vi "Open Channel.vi"(6 "Open All (False)":bool, 7 "Channel List":string, 8 "error in (no error)":errorcluster, 11 "VISA resource name":refnum<visa-resource-name>) -> (0 "error out":errorcluster, 3 "VISA resource name out":refnum<visa-resource-name>)   [LabVIEW 2018, in "Keithley 3706.lvlib"]
uses:
  <instrlib>/Keithley 3706/Keithley 3706.lvlib
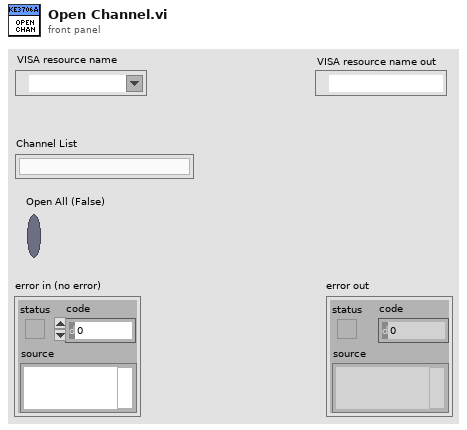
[diagram p1: front panel]
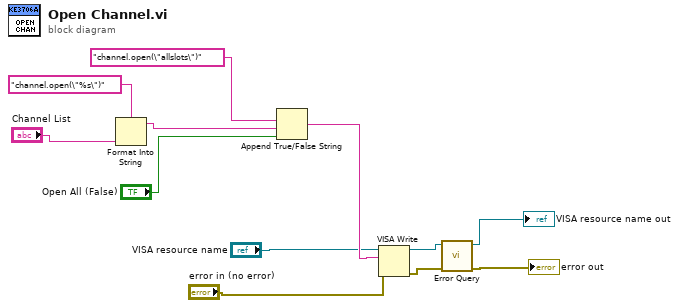
[diagram p0: block diagram]
diagram:
  n1 = Format Into String(format string="channel.open(\"%s\")", "Channel List") -> (resulting string=w10:string)  [unwired: 2 in, 1 out]
  n2 = Append True/False String(1:"Open All (False)", 2:w10, 3:"channel.open(\"allslots\")") -> (0:w7:string)  [unwired: 1 in]
  n3 = VISA Write(VISA resource name="VISA resource name", write buffer=w7, error in (no error)="error in (no error)") -> (VISA resource name out=w4:refnum<visa-resource-name>, error out=w3:errorcluster)  [unwired: 1 out]
  n4 = call <instrlib>:"Error Query.vi"("error in (no error)"=w3, "VISA resource name"=w4) -> ("error out"=→"error out":errorcluster, "VISA resource name output"=→"VISA resource name out":refnum<visa-resource-name>)  [unwired: 6 in, 2 out]
